vi "添加启动项.vi"(8 "error in (no error)":errorcluster caption="错误输入（无错误）", 11 "启动文件路径":path) -> (0 "error out":errorcluster caption="错误输出", 3 "添加成功标记":bool)   [LabVIEW 2016]
uses:
  <vilib>/registry/registry.llb/Registry RtKey.ctl
  <vilib>/registry/registry.llb/Write Registry Value Simple STR.vi
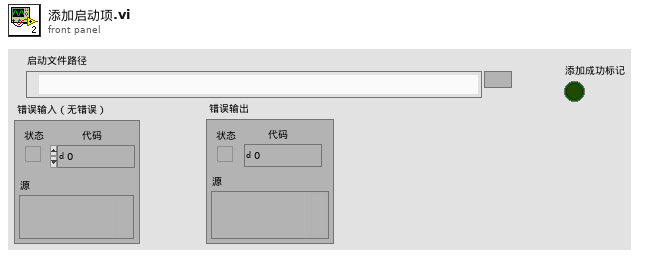
[diagram p1: front panel]
types:
  T1 = typedef "Registry RtKey.ctl" = enum32{"HKEY_CLASSES_ROOT", "HKEY_CURRENT_USER", "HKEY_LOCAL_MACHINE", "HKEY_USERS", "HKEY_PERFORMANCE_DATA", "HKEY_CURRENT_CONFIG", "HKEY_DYN_DATA"}
  T2 = typedef "Registry refnum.ctl" = refnum<k1>
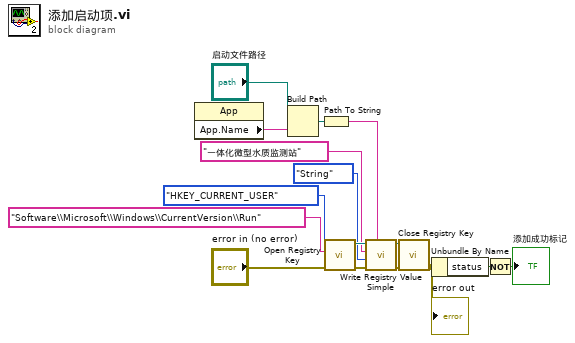
[diagram p0: block diagram]
diagram:
  n1 = property class="App"() -> ("App.Name"=w2:string)  [unwired: 2 in, 2 out]
  n2 = Build Path(base path="启动文件路径", name or relative path=w2) -> (appended path=w1:path)
  n3 = Path To String(path=w1) -> (string=w5:string)
  n4 = call <vilib>:"Open Registry Key.vi"("error in (no error)"="error in (no error)", "subkey"="Software\\Microsoft\\Windows\\CurrentVersion\\Run", "root key (HKEY_LOCAL_MACHINE)"=Registry_RtKey."HKEY_CURRENT_USER") -> ("error out"=w13:errorcluster, "refnum out"=w12:T2)  [unwired: 7 in]
  n5 = call-poly <vilib>:"Write Registry Value Simple.vi"("String/Binary data"=w5, "error in (no error)"=w13, "simple data type"=enum16{"String", "Binary", "DWORD"}."String", "value"="一体化微型水质监测站", "refnum"=w12) -> ("error out"=w15:errorcluster, "refnum out"=w14:T2)  [unwired: 3 in]
  n6 = call <vilib>:"Close Registry Key.vi"("error in (no error)"=w15, "refnum"=w14) -> ("error out"=w7:errorcluster)  [unwired: 5 in]
  "error out" <- w7
  n7 = Unbundle By Name(w7) -> ("status"=w6:bool)
  n8 = Not(x=w6) -> (.not. x?=→"添加成功标记":bool)
